vi "Disconnect.vi"(8 "error in (no error)":errorcluster, 11 "Telnet V2 in":refnum<class "Telnet V2.lvclass">) -> (0 "error out":errorcluster, 3 "Telnet V2 out":refnum<class "Telnet V2.lvclass">)   [LabVIEW 2018, in "Telnet V2.lvlib" / "Telnet V2.lvclass"]
uses:
  Telnet V2.lvclass
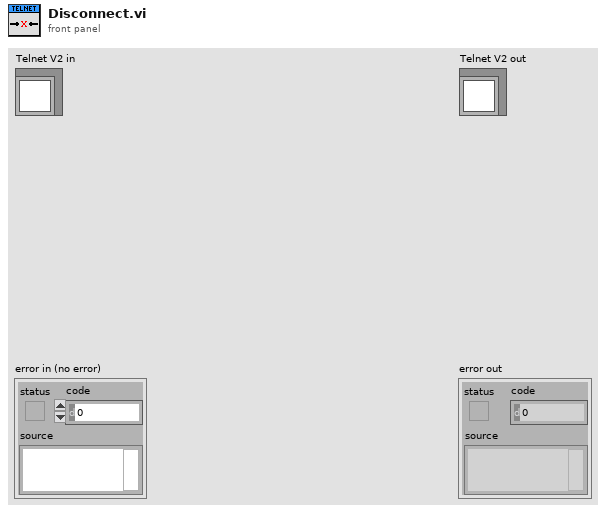
[diagram p1: front panel]
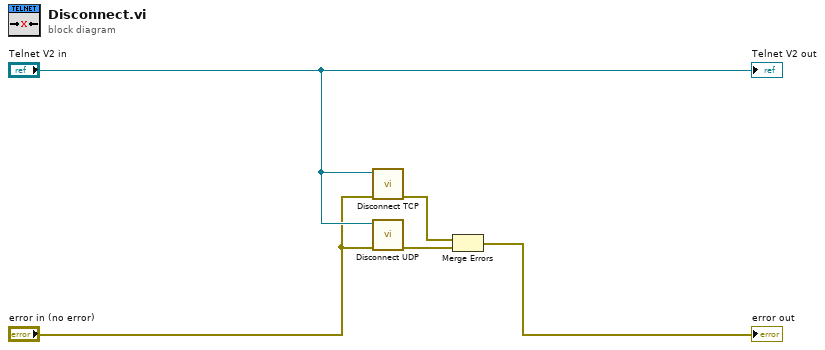
[diagram p0: block diagram]
diagram:
  n1 = call-dynamic "Disconnect TCP.vi"("error in (no error)"="error in (no error)", "Telnet V2 in"="Telnet V2 in") -> ("error out"=w2:errorcluster)  [unwired: 8 in, 1 out]
  n2 = call-dynamic "Disconnect UDP.vi"("error in (no error)"="error in (no error)", "Telnet V2 in"="Telnet V2 in") -> ("error out"=w3:errorcluster)  [unwired: 8 in, 1 out]
  n3 = Merge Errors(w2, w3) -> (→"error out":errorcluster)
  "Telnet V2 out" <- "Telnet V2 in"
